vi "Write header into the image.vi"(8 "error in (no error)":errorcluster, 11 "Save Image in":refnum<class "Save Image.lvclass">) -> (0 "error out":errorcluster, 3 "Save Image out":refnum<class "Save Image.lvclass">)   [LabVIEW 2018, in "Save Image.lvclass"]
uses:
  Save Image.lvclass
  Save Image.lvclass/Save Image.ctl
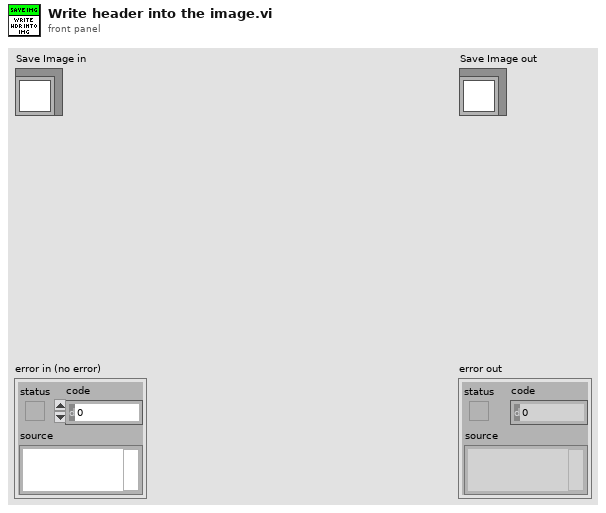
[diagram p1: front panel]
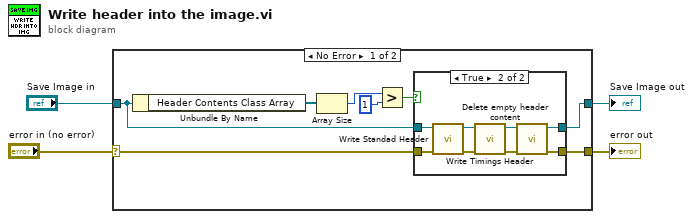
[diagram p0: block diagram]
diagram:
  n1 = case shown="No Error" "error in (no error)" {
    selector: "error in (no error)" -> [w5 w24]
    tunnel: [w9 w24] -> w3
    tunnel: [w7 w23] -> w1
    tunnel: "Save Image in" -> [w8 w23]
    frame No Error {
      n2 = Unbundle By Name(w8) -> ("Header Contents Class Array"=w6:refnum<class "Simulated_Header.lvclass">[])
      n3 = Array Size(array=w6) -> (size(s)=w12:i32)
      n4 = Greater?(x=w12, y=1) -> (0:w10:bool)
      n5 = case shown="True" w10 {
        tunnel: w5 -> [w14 w21]
        tunnel: [w14 w16] -> w9
        tunnel: w8 -> [w13 w22]
        tunnel: [w13 w15] -> w7
        frame False {
        }
        frame True {
          n6 = call "Write Standad Header.vi"("error in (no error)"=w21, "Save Image in"=w22) -> ("error out"=w19:errorcluster, "Save Image out"=w20:refnum<class "Save Image.lvclass">)  [unwired: 8 in]
          n7 = call "Write Timings Header.vi"("error in (no error)"=w19, "Save Image in"=w20) -> ("error out"=w17:errorcluster, "Save Image out"=w18:refnum<class "Save Image.lvclass">)  [unwired: 8 in]
          n8 = call "Delete empty header content.vi"("error in (no error)"=w17, "Save Image in"=w18) -> ("error out"=w16:errorcluster, "Save Image out"=w15:refnum<class "Save Image.lvclass">)  [unwired: 8 in]
        }
      }
    }
    frame Error {
    }
  }
  "error out" <- w3
  "Save Image out" <- w1
